vi "Dialog GraphSetting (Chart).vi"(11 "波形チャートref(in)":refnum<vi>) -> ()   [LabVIEW 2014]
uses:
  TypeDef/GraphSetting Appearance.ctl
  TypeDef/GraphSetting Plot.ctl
  SupportVIs/GraphSetting Scale.ctl
  TypeDef/GraphSetting DisplayFormatType.ctl
  TypeDef/GraphSetting All.ctl
  TypeDef/GraphSetting Command.ctl
  Lib/Event/Write User Event (Array).vi
  <vilib>/Utility/xml.llb/Write to XML File(string).vi
  <vilib>/Utility/xml.llb/Read From XML File(string).vi
panel:
  in  "ファイル読込":bool
  in  "ファイル保存":bool
  in  "タブ制御器":enum32{"外観", "スケール", "プロット"}(tab)
  in  "外観":T1
  in  "Yスケール選択":u16(ring) items=["振幅"]
  in  "スケール(Y軸)":T2
  in  "スケール(X軸)":T2
  in  "Xスケール選択":u16(ring) items=["時間"]
  in  "プロット":T4 {"Yスケール" items=["振幅"]; "Xスケール" items=["時間"]; "プロット補間" max=5 step=1; "ポイントスタイル" max=16 step=1; "太さ" max=5 step=1; "ラインスタイル" max=4 step=1}
  in  "プロット選択":u16(ring) items=["正弦波", "プロット1"]
  in  "停止ボタン":bool
  # "欄外、パラメータ"
  # "スケールのスタイルとカラー"
  # "スケール係数"
  # "スケールのスタイルとカラー"
  # "スケールのスタイルとカラー"
  # "スケール係数"
  # "スケールのスタイルとカラー"
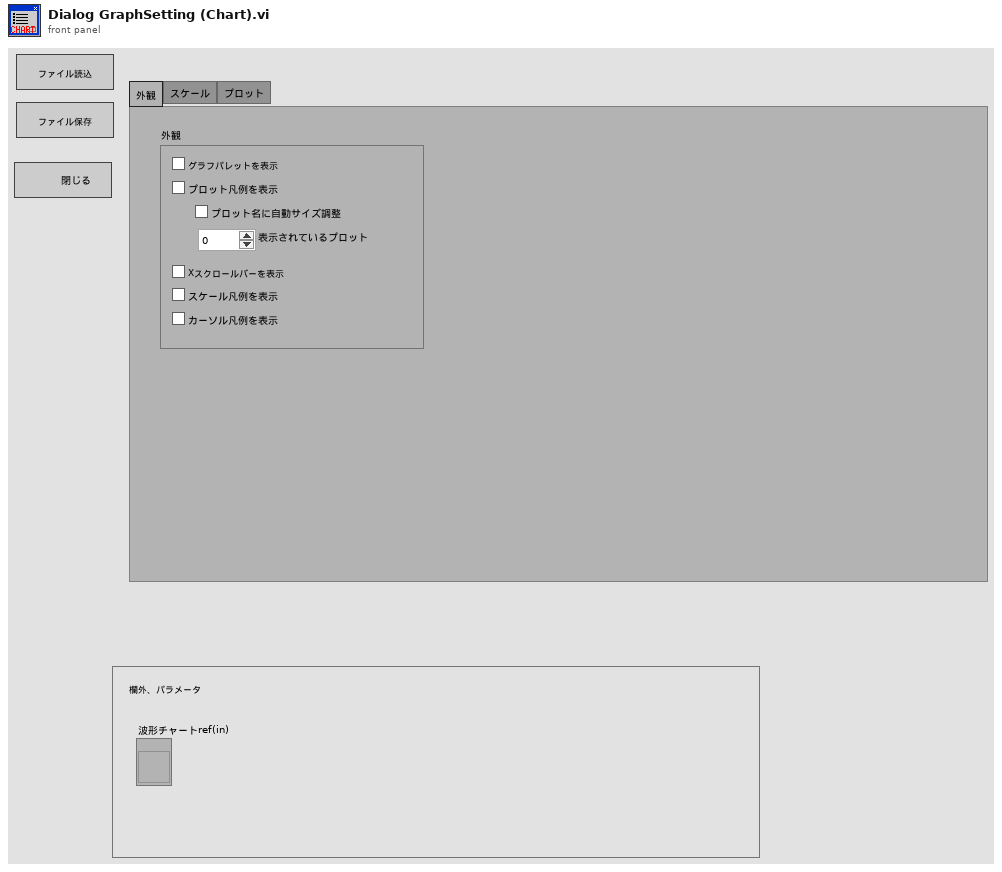
[diagram p1: front panel]
types:
  T1 = typedef "GraphSetting Appearance.ctl" = cluster{"グラフパレットを表示":bool, "プロット凡例を表示":bool, "プロット名に自動サイズ調整":bool, "表示されているプロット":u32, "Xスクロールバーを表示":bool, "スケール凡例を表示":bool, "カーソル凡例を表示":bool}
  T2 = typedef "GraphSetting Scale.ctl" = cluster{"名前":string, "スケールラベルを表示":bool, "スケールを表示":bool, "ログ":bool, "反転":bool, "自動スケール":bool, "最小":dbl, "最大":dbl, "オフセット":dbl, "乗数":dbl, "主目盛り":u32, "補助目盛り":u32, "マーカテキスト":u32, "主グリッド":u32, "補助グリッド":u32, "タイプ":T3, "小数点以下桁数":u8}
  T3 = typedef "GraphSetting DisplayFormatType.ctl" = enum8{"浮動小数点", "科学", "工学", "バイナリ", "８進数", "１６進数", "相対時間", "時間と日時", "SI"}
  T4 = typedef "GraphSetting Plot.ctl" = cluster{"名前":string, "表示":bool, "ラインスタイル":u8, "太さ":u8, "ポイントスタイル":u8, "プロット補間":u8, "ラインカラー":u32, "ポイント/塗りつぶし":u32, "Xスケール":u16, "Yスケール":u16}
  T5 = typedef "GraphSetting All.ctl" = cluster{"外観":T1, "スケールX[]":T2[], "スケールY[]":T2[], "プロット[]":T4[]}
  T6 = typedef "GraphSetting Command.ctl" = enum16{"Get(ref->ctl)", "Set(ctl->ref)"}
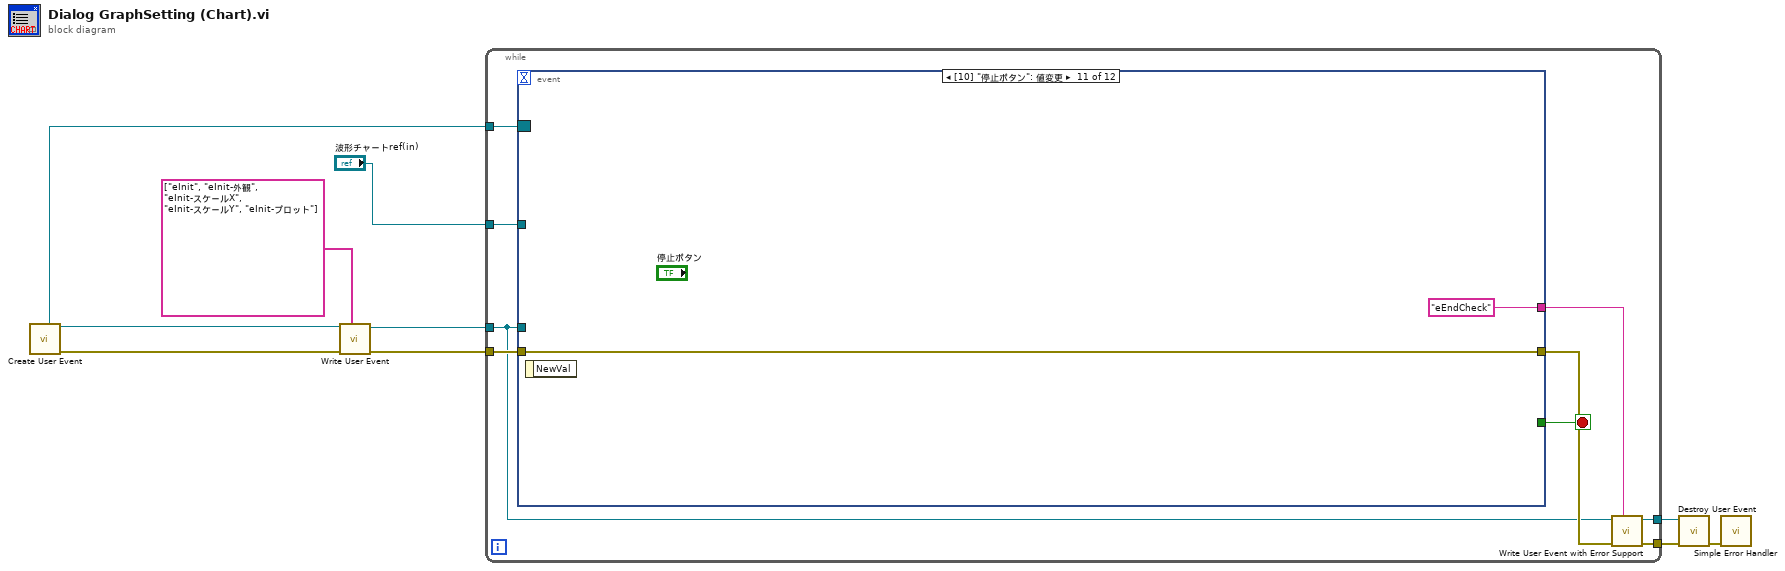
[diagram p0: block diagram]
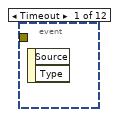
[diagram p2: hidden frame]
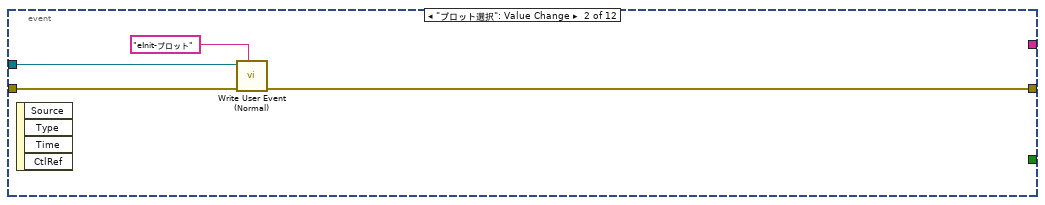
[diagram p3: hidden frame]
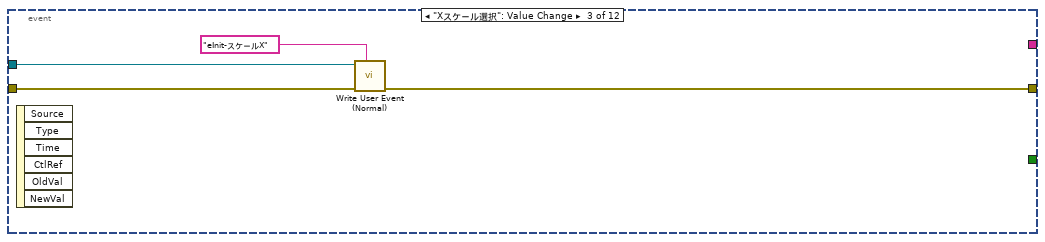
[diagram p4: hidden frame]
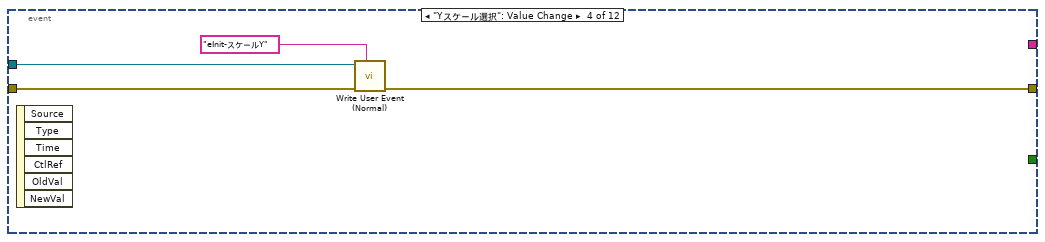
[diagram p5: hidden frame]
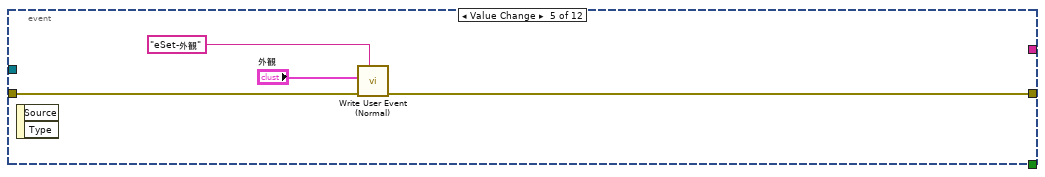
[diagram p6: hidden frame]
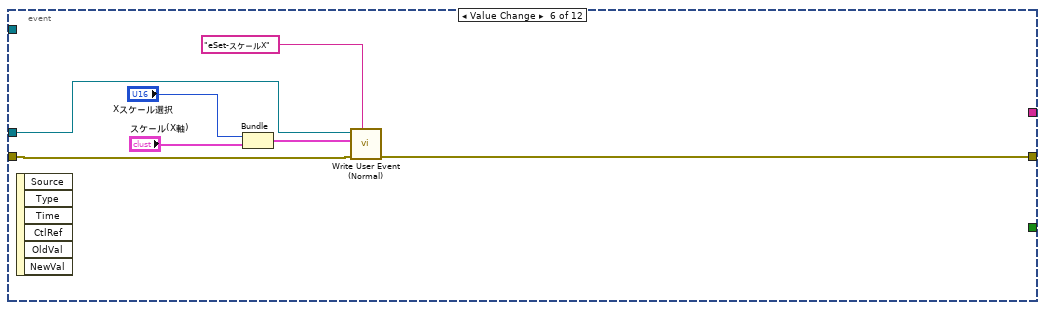
[diagram p7: hidden frame]
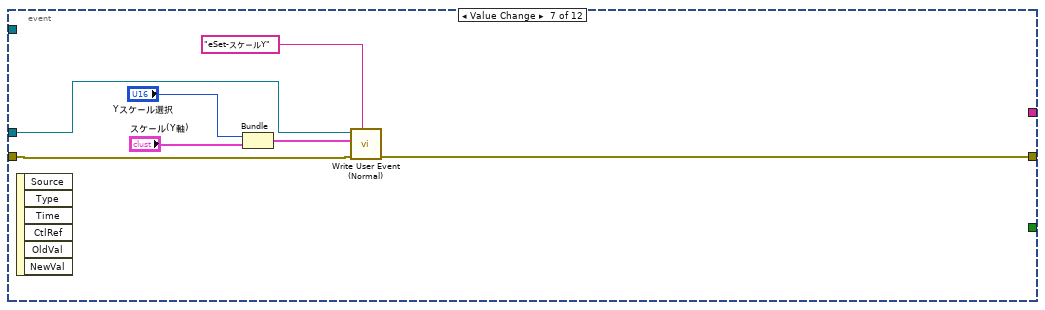
[diagram p8: hidden frame]
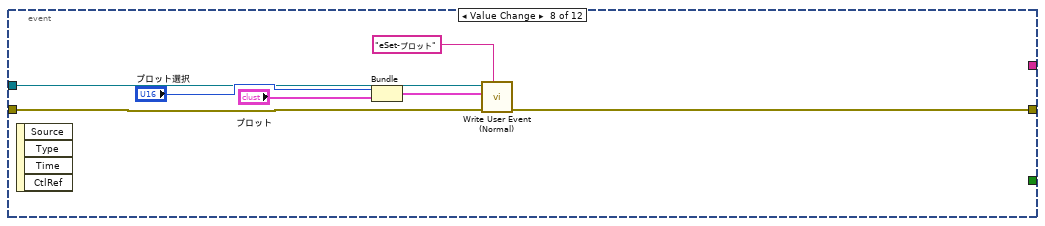
[diagram p9: hidden frame]
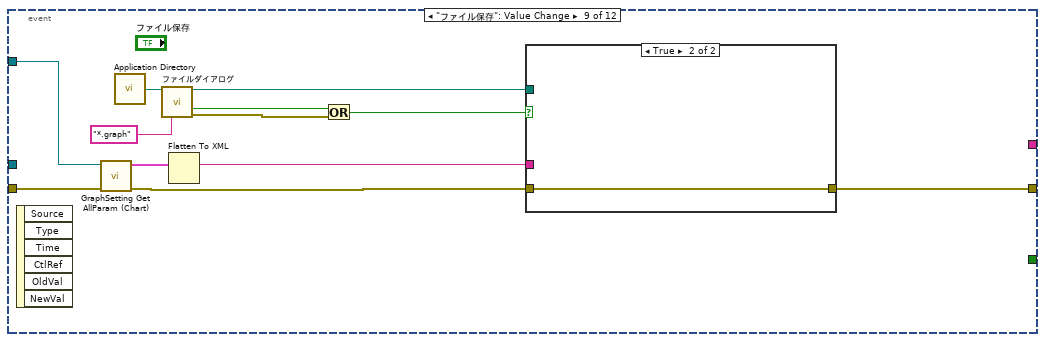
[diagram p10: hidden frame]
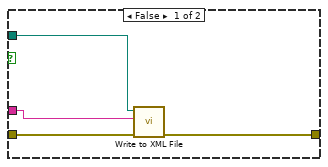
[diagram p11: hidden frame]
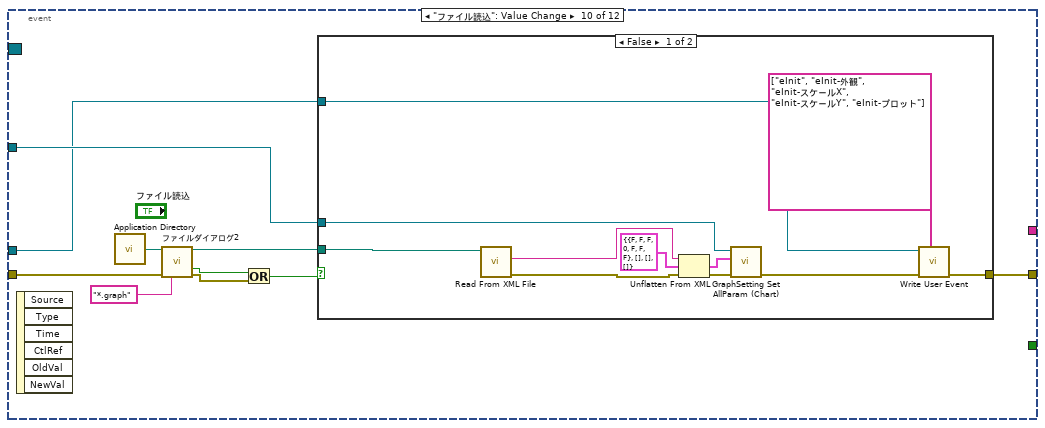
[diagram p12: hidden frame]
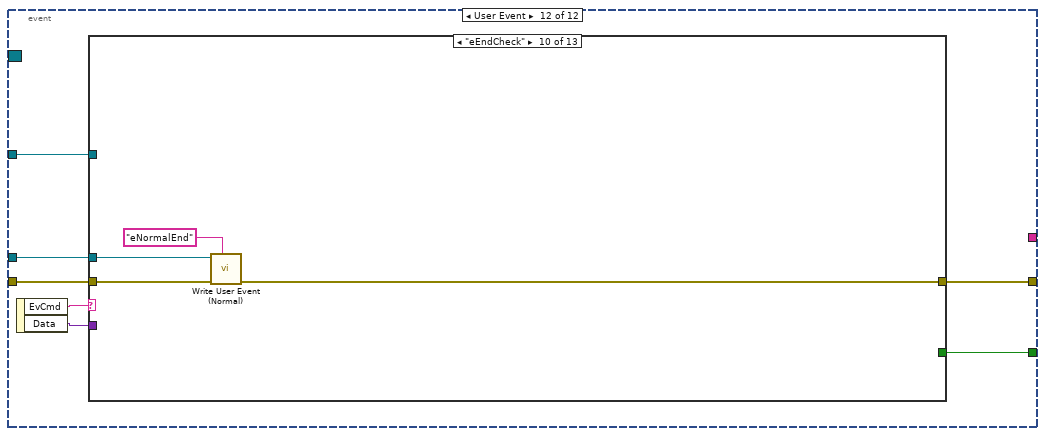
[diagram p14: hidden frame]
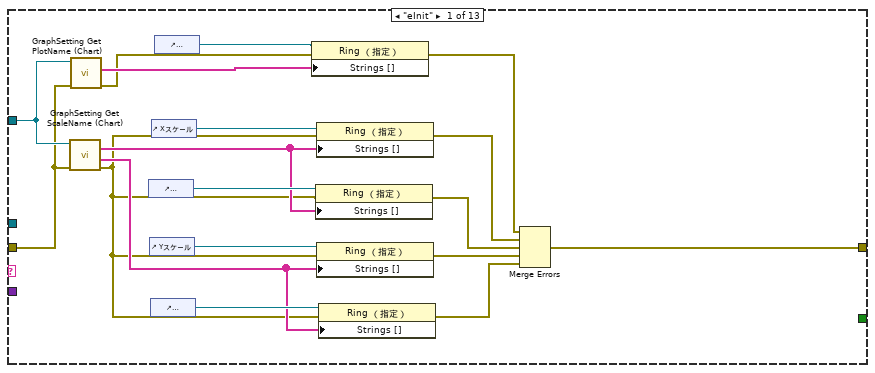
[diagram p15: hidden frame]
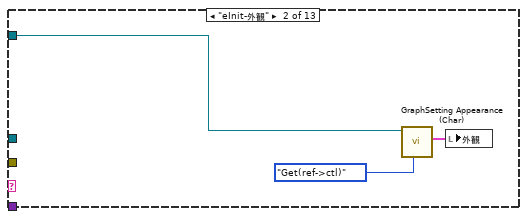
[diagram p16: hidden frame]
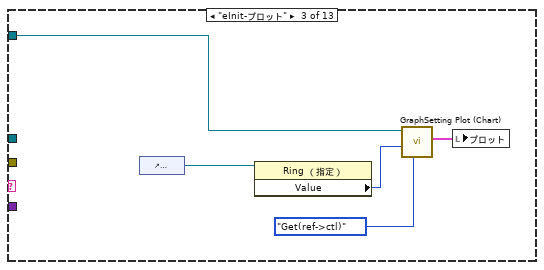
[diagram p17: hidden frame]
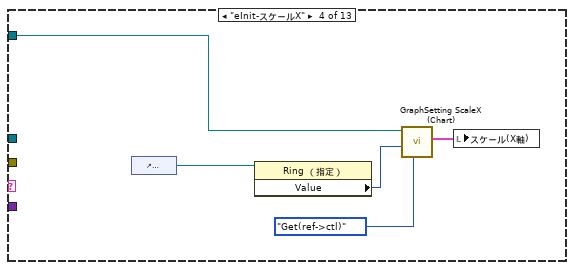
[diagram p18: hidden frame]
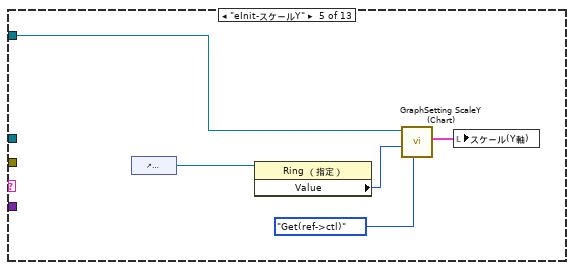
[diagram p19: hidden frame]
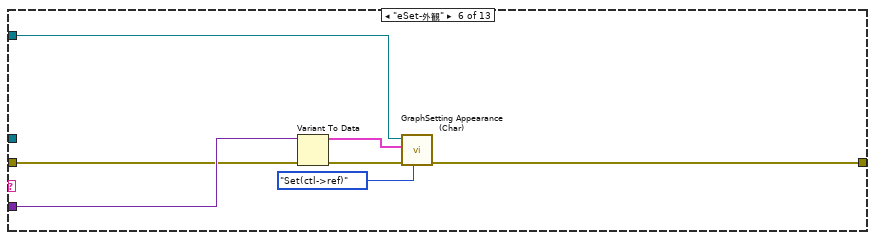
[diagram p20: hidden frame]
diagram:
  n1 = call "Create User Event.vi"() -> ("error out"=w8:errorcluster, "User Event"=w9:refnum<user-event>, "Event Registration Refnum"=w10:refnum<event-registration>)  [unwired: 9 in]
  n2 = call-poly "Write User Event.vi"("EvCmd[]"=string[] ["eInit", "eInit-外観", "eInit-スケールX", "eInit-スケールY", "eInit-プロット"], "エラー入力（エラーなし）"=w8, "ユーザイベント入力"=w9) -> ("エラー出力"=w4:errorcluster, "ユーザイベント出力"=w5:refnum<user-event>)  [unwired: 7 in]
  n3 = while {
    tunnel: w4 -> [w18]
    tunnel: w10 -> [w19]
    tunnel: [w15] -> w7
    tunnel: w5 -> [w11]
    tunnel: "波形チャートref(in)" -> [w17]
    tunnel: [w12] -> w2
    stop <- w13 stop-if-true
    n4 = event shown="[10] \"停止ボタン\": 値変更" {
      selector: w19 -> [_ _ _ _ _ _ _ _ _ _ _ _]
      dyn-events: _ -> [_ _ _ _ _ _ _ _ _ _ _ _]
      timeout: _ -> [_ _ _ _ _ _ _ _ _ _ _ _]
      tunnel: [_ _ _ _ _ _ _ _ _ _ _ w99] -> w13
      tunnel: [_ w21 w25 w28 w32 w37 w44 w51 w60 w78 w95 w100] -> w16
      tunnel: w18 -> [_ w22 w27 w30 w33 w36 w45 w52 w67 w81 w95 w101]
      tunnel: w11 -> [_ w23 w26 w29 _ w40 w46 w53 _ w77 _ w98]
      tunnel: w17 -> [_ _ _ _ _ _ _ _ w68 w79 _ w97]
      tunnel: [_ _ _ _ _ _ _ _ _ _ "eEndCheck" _] -> w14
      event Timeout {
        n5 = event-data() -> ()  [unwired: 1 in, 2 out]
      }
      event "プロット選択": Value Change {
        n6 = event-data() -> ()  [unwired: 1 in, 4 out]
        n7 = call "Write User Event (Normal).vi"("EvCmd"="eInit-プロット", "エラー入力（エラーなし）"=w22, "ユーザイベント入力"=w23) -> ("エラー出力"=w21:errorcluster)  [unwired: 7 in, 1 out]
      }
      event "Xスケール選択": Value Change {
        n8 = event-data() -> ()  [unwired: 1 in, 6 out]
        n9 = call "Write User Event (Normal).vi"("EvCmd"="eInit-スケールX", "エラー入力（エラーなし）"=w27, "ユーザイベント入力"=w26) -> ("エラー出力"=w25:errorcluster)  [unwired: 7 in, 1 out]
      }
      event "Yスケール選択": Value Change {
        n10 = event-data() -> ()  [unwired: 1 in, 6 out]
        n11 = call "Write User Event (Normal).vi"("EvCmd"="eInit-スケールY", "エラー入力（エラーなし）"=w30, "ユーザイベント入力"=w29) -> ("エラー出力"=w28:errorcluster)  [unwired: 7 in, 1 out]
      }
      event Value Change {
        n12 = event-data() -> ()  [unwired: 1 in, 2 out]
        n13 = call "Write User Event (Normal).vi"("EvCmd"="eSet-外観", "エラー入力（エラーなし）"=w33, "データ"="外観") -> ("エラー出力"=w32:errorcluster)  [unwired: 7 in, 1 out]
      }
      event Value Change {
        n14 = event-data() -> ()  [unwired: 1 in, 6 out]
        n15 = Bundle("Xスケール選択"="Xスケール選択", "スケール(X軸)"="スケール(X軸)") -> (w41:cluster{"Xスケール選択":u16, "スケール(X軸)":T2})  [unwired: 1 in]
        n16 = call "Write User Event (Normal).vi"("EvCmd"="eSet-スケールX", "エラー入力（エラーなし）"=w36, "データ"=w41, "ユーザイベント入力"=w40) -> ("エラー出力"=w37:errorcluster)  [unwired: 6 in, 1 out]
      }
      event Value Change {
        n17 = event-data() -> ()  [unwired: 1 in, 6 out]
        n18 = Bundle("Yスケール選択"="Yスケール選択", "スケール(Y軸)"="スケール(Y軸)") -> (w47:cluster{"Yスケール選択":u16, "スケール(Y軸)":T2})  [unwired: 1 in]
        n19 = call "Write User Event (Normal).vi"("EvCmd"="eSet-スケールY", "エラー入力（エラーなし）"=w45, "データ"=w47, "ユーザイベント入力"=w46) -> ("エラー出力"=w44:errorcluster)  [unwired: 6 in, 1 out]
      }
      event Value Change {
        n20 = event-data() -> ()  [unwired: 1 in, 4 out]
        n21 = Bundle("プロット選択"="プロット選択", "プロット"="プロット") -> (w54:cluster{"プロット選択":u16, "プロット":T4})  [unwired: 1 in]
        n22 = call "Write User Event (Normal).vi"("EvCmd"="eSet-プロット", "エラー入力（エラーなし）"=w52, "データ"=w54, "ユーザイベント入力"=w53) -> ("エラー出力"=w51:errorcluster)  [unwired: 6 in, 1 out]
      }
      event "ファイル保存": Value Change {
        n23 = event-data() -> ()  [unwired: 1 in, 6 out]
        n24 = call "GraphSetting Get AllParam (Chart).vi"("エラー入力（エラーなし）"=w67, "WaveformChart入力"=w68) -> ("エラー出力"=w62:errorcluster, "クラスタ"=w61:cluster{"外観(out)":T1, T2[], T2[], T4[]})  [unwired: 8 in]
        n25 = call <vilib>:"Application Directory.vi"() -> ("Application Directory"=w65:path)
        n26 = call "ファイルダイアログ"("start path"=w65, "pattern (all files)"="*.graph") -> ("selected path"=w63:path, "cancelled"=w59:bool, "error out"=w58:errorcluster)  [unwired: 10 in, 1 out]
        n27 = Flatten To XML(anything=w61) -> (xml string=w64:string)
        n28 = Or(x=w59, y=w58) -> (x .or. y?=w57:bool)
        n29 = case shown="TRUE" w57 {
          tunnel: w63 -> [w72 _]
          tunnel: w64 -> [w71 _]
          tunnel: w62 -> [w69 w73]
          tunnel: [w70 w73] -> w60
          frame False {
            n30 = call-poly <vilib>:"Write to XML File.vi"("error in (no error)"=w69, "XML Input"=w71, "XML File Path"=w72) -> ("error out"=w70:errorcluster)  [unwired: 6 in, 2 out]
          }
          frame True {
          }
        }
      }
      event "ファイル読込": Value Change {
        n31 = event-data() -> ()  [unwired: 1 in, 6 out]
        n32 = call <vilib>:"Application Directory.vi"() -> ("Application Directory"=w83:path)
        n33 = call "ファイルダイアログ2"("start path"=w83, "error in"=w81, "pattern (all files)"="*.graph") -> ("selected path"=w80:path, "cancelled"=w75:bool, "error out"=w74:errorcluster)  [unwired: 9 in, 1 out]
        n34 = Or(x=w75, y=w74) -> (x .or. y?=w76:bool)
        n35 = case shown="FALSE" w76 {
          tunnel: w80 -> [w92 _]
          tunnel: w79 -> [w88 _]
          tunnel: [w85 _] -> w78
          tunnel: w77 -> [w87 _]
          frame False {
            n36 = call-poly <vilib>:"Read From XML File.vi"("XML File Path"=w92) -> ("error out"=w91:errorcluster, "XML Elements"=w93:string)  [unwired: 8 in, 1 out]
            n37 = Unflatten From XML(xml string=w93, type=T5 {"外観"={"グラフパレットを表示"=FALSE, "プロット凡例を表示"=FALSE, "プロット名に自動サイズ調整"=FALSE, "表示されているプロット"=0, "Xスクロールバーを表示"=FALSE, "スケール凡例を表示"=FALSE, "カーソル凡例を表示"=FALSE}, "スケールX[]"=[], "スケールY[]"=[], "プロット[]"=[]} ("出力クラスタ"), error in (no error)=w91) -> (value=w90:T5, error out=w89:errorcluster)
            n38 = call "GraphSetting Set AllParam (Chart).vi"("error in (no error)"=w89, "Chartグラフパラメータ"=w90, "波形チャートref(in)"=w88) -> ("error out"=w86:errorcluster)  [unwired: 8 in]
            n39 = call-poly "Write User Event.vi"("EvCmd[]"=string[] ["eInit", "eInit-外観", "eInit-スケールX", "eInit-スケールY", "eInit-プロット"], "エラー入力（エラーなし）"=w86, "ユーザイベント入力"=w87) -> ("エラー出力"=w85:errorcluster)  [unwired: 7 in, 1 out]
          }
          frame True {
          }
        }
      }
      event "停止ボタン": Value Change {
        n40 = event-data() -> ()  [unwired: 1 in, 1 out]
      }
      event User Event {
        n41 = event-data() -> ("EvCmd"=w103:string, "Data"=w102:variant)  [unwired: 1 in]
        n42 = case shown="\"eEndCheck\"" w103 {
          selector: w103 -> [_ _ _ _ _ _ _ _ _ _ _ _ w187]
          tunnel: w102 -> [_ _ _ _ _ w144 w152 w163 w173 _ _ w186 _]
          tunnel: w101 -> [w113 _ _ _ _ w142 w154 w162 w172 w177 w181 w184 _]
          tunnel: [w104 _ _ _ _ w140 w147 w156 w166 w176 w181 _ _] -> w100
          tunnel: [_ _ _ _ _ _ _ _ _ _ TRUE TRUE _] -> w99
          tunnel: w98 -> [_ _ _ _ _ _ _ _ _ w179 _ _ _]
          tunnel: w97 -> [w116 w124 w129 w134 w139 w145 w148 w160 w170 _ _ _ _]
          frame "eInit" {
            n43 = call "GraphSetting Get ScaleName (Chart).vi"("error in (no error)"=w113, "波形チャートref(in)"=w116) -> ("error out"=w110:errorcluster, "Y軸名称[]"=w112:string[], "X軸名称[]"=w119:string[])  [unwired: 7 in]
            n44 = call "GraphSetting Get PlotName (Chart).vi"("error in (no error)"=w113, "波形チャートref(in)"=w116) -> ("error out"=w111:errorcluster, "プロット名称[]"=w114:string[])  [unwired: 8 in]
            n45 = control-ref of="Xスケール選択"() -> (w120:refnum<vi>)
            n46 = control-ref of="Yスケール"() -> (w117:refnum<vi>)
            n47 = control-ref of="Yスケール選択"() -> (w118:refnum<vi>)
            n48 = control-ref of="Xスケール"() -> (w121:refnum<vi>)
            n49 = control-ref of="プロット選択"() -> (w115:refnum<vi>)
            n50 = property class="Ring （指定）"(reference=w115, error in=w111, "Strings []"=w114) -> (error out=w109:errorcluster)  [unwired: 1 out]
            n51 = property class="Ring （指定）"(reference=w120, error in=w110, "Strings []"=w119) -> (error out=w107:errorcluster)  [unwired: 1 out]
            n52 = property class="Ring （指定）"(reference=w121, error in=w110, "Strings []"=w119) -> (error out=w108:errorcluster)  [unwired: 1 out]
            n53 = property class="Ring （指定）"(reference=w117, error in=w110, "Strings []"=w112) -> (error out=w106:errorcluster)  [unwired: 1 out]
            n54 = property class="Ring （指定）"(reference=w118, error in=w110, "Strings []"=w112) -> (error out=w105:errorcluster)  [unwired: 1 out]
            n55 = Merge Errors(w109, w108, w107, w106, w105) -> (w104:errorcluster)
          }
          frame "eInit-外観" {
            n56 = call "GraphSetting Appearance (Char).vi"("コマンド"=GraphSetting_Command."Get(ref->ctl)", "WaveformChart入力"=w124) -> ("外観(out)"=w123:T1)  [unwired: 8 in, 1 out]
            n57 = local write "外観"(w123) -> ()
          }
          frame "eInit-プロット" {
            n58 = control-ref of="プロット選択"() -> (w128:refnum<vi>)
            n59 = property class="Ring （指定）"(reference=w128) -> ("Value"=w127:u16)  [unwired: 1 in, 2 out]
            n60 = call "GraphSetting Plot (Chart).vi"("コマンド"=GraphSetting_Command."Get(ref->ctl)", "アクティブプロット"=w127, "波形チャートref(in)"=w129) -> ("プロット(out)"=w125:T4)  [unwired: 7 in, 1 out]
            n61 = local write "プロット"(w125) -> ()
          }
          frame "eInit-スケールX" {
            n62 = control-ref of="Xスケール選択"() -> (w133:refnum<vi>)
            n63 = property class="Ring （指定）"(reference=w133) -> ("Value"=w132:u16)  [unwired: 1 in, 2 out]
            n64 = call "GraphSetting ScaleX (Chart).vi"("コマンド"=GraphSetting_Command."Get(ref->ctl)", "アクティブスケール(X)"=w132, "波形チャートref(in)"=w134) -> ("スケール(out)"=w130:T2)  [unwired: 7 in, 1 out]
            n65 = local write "スケール(X軸)"(w130) -> ()
          }
          frame "eInit-スケールY" {
            n66 = control-ref of="Yスケール選択"() -> (w138:refnum<vi>)
            n67 = property class="Ring （指定）"(reference=w138) -> ("Value"=w137:u16)  [unwired: 1 in, 2 out]
            n68 = call "GraphSetting ScaleY (Chart).vi"("コマンド"=GraphSetting_Command."Get(ref->ctl)", "アクティブスケールY"=w137, "波形チャートref(in)"=w139) -> ("スケール(out)"=w135:T2)  [unwired: 7 in, 1 out]
            n69 = local write "スケール(Y軸)"(w135) -> ()
          }
          frame "eSet-外観" {
            n70 = Variant To Data(error in=w142, Variant=w144) -> (data=w143:T1, error out=w141:errorcluster)  [unwired: 1 in]
            n71 = call "GraphSetting Appearance (Char).vi"("コマンド"=GraphSetting_Command."Set(ctl->ref)", "error in (no error)"=w141, "外観(in)"=w143, "WaveformChart入力"=w145) -> ("error out"=w140:errorcluster)  [unwired: 6 in, 1 out]
          }
          frame "eSet-スケールX" {
            n72 = Variant To Data(type=cluster{"Xスケール選択":u16, "スケール(X軸)":T2} {"Xスケール選択"=0, "スケール(X軸)"={"名前"="", "スケールラベルを表示"=FALSE, "スケールを表示"=FALSE, "ログ"=FALSE, "反転"=FALSE, "自動スケール"=FALSE, "最小"=0.0, "最大"=0.0, "オフセット"=0.0, "乗数"=0.0, "主目盛り"=0, "補助目盛り"=0, "マーカテキスト"=0, "主グリッド"=0, "補助グリッド"=0, "タイプ"=enum."浮動小数点", "小数点以下桁数"=0}} ("出力クラスタ"), Variant=w152) -> (data=w151:cluster{"Xスケール選択":u16, "スケール(X軸)":T2})  [unwired: 1 in, 1 out]
            n73 = Unbundle(w151) -> ("Xスケール選択"=w149:u16, "スケール(X軸)"=w150:T2)
            n74 = call "GraphSetting ScaleX (Chart).vi"("コマンド"=GraphSetting_Command."Set(ctl->ref)", "error in (no error)"=w154, "アクティブスケール(X)"=w149, "スケール(in)"=w150, "波形チャートref(in)"=w148) -> ("error out"=w147:errorcluster)  [unwired: 5 in, 1 out]
          }
          frame "eSet-スケールY" {
            n75 = Variant To Data(error in=w162, type=cluster{"Xスケール選択":u16, "スケール(X軸)":T2} {"Xスケール選択"=0, "スケール(X軸)"={"名前"="", "スケールラベルを表示"=FALSE, "スケールを表示"=FALSE, "ログ"=FALSE, "反転"=FALSE, "自動スケール"=FALSE, "最小"=0.0, "最大"=0.0, "オフセット"=0.0, "乗数"=0.0, "主目盛り"=0, "補助目盛り"=0, "マーカテキスト"=0, "主グリッド"=0, "補助グリッド"=0, "タイプ"=enum."浮動小数点", "小数点以下桁数"=0}} ("出力クラスタ"), Variant=w163) -> (data=w161:cluster{"Xスケール選択":u16, "スケール(X軸)":T2}, error out=w157:errorcluster)
            n76 = Unbundle(w161) -> ("Xスケール選択"=w158:u16, "スケール(X軸)"=w159:T2)
            n77 = call "GraphSetting ScaleY (Chart).vi"("コマンド"=GraphSetting_Command."Set(ctl->ref)", "error in (no error)"=w157, "アクティブスケールY"=w158, "スケール(in)"=w159, "波形チャートref(in)"=w160) -> ("error out"=w156:errorcluster)  [unwired: 5 in, 1 out]
          }
          frame "eSet-プロット" {
            n78 = Variant To Data(error in=w172, type=cluster{"プロット選択":u16, "プロット":T4} {"プロット選択"=0, "プロット"={"名前"="", "表示"=FALSE, "ラインスタイル"=0, "太さ"=0, "ポイントスタイル"=0, "プロット補間"=0, "ラインカラー"=0, "ポイント/塗りつぶし"=0, "Xスケール"=0, "Yスケール"=0}} ("出力クラスタ"), Variant=w173) -> (data=w171:cluster{"プロット選択":u16, "プロット":T4}, error out=w169:errorcluster)
            n79 = Unbundle(w171) -> ("プロット選択"=w168:u16, "プロット"=w167:T4)
            n80 = call "GraphSetting Plot (Chart).vi"("コマンド"=GraphSetting_Command."Set(ctl->ref)", "error in (no error)"=w169, "アクティブプロット"=w168, "プロット(in)"=w167, "波形チャートref(in)"=w170) -> ("error out"=w166:errorcluster)  [unwired: 5 in, 1 out]
          }
          frame "eEndCheck" {
            n81 = call "Write User Event (Normal).vi"("EvCmd"="eNormalEnd", "エラー入力（エラーなし）"=w177, "ユーザイベント入力"=w179) -> ("エラー出力"=w176:errorcluster)  [unwired: 7 in, 1 out]
          }
          frame "eNormalEnd" {
          }
          frame "eErrorEnd" {
            n82 = Variant To Data(error in=w184, type=errorcluster {"status"=FALSE, "code"=0, "source"=""} ("エラー定数"), Variant=w186) -> (data=w183:errorcluster)  [unwired: 1 out]
            n83 = call <vilib>:"Simple Error Handler.vi"("error in (no error)"=w183) -> ()  [unwired: 4 in, 5 out]
          }
          frame Default {
            n84 = call "DialogProgramError.vi"("エラー内容"="ユーザイベント例外" ("エラー詳細"), "エラー詳細"=w187) -> ()  [unwired: 9 in, 1 out]
          }
        }
      }
    }
    n85 = call "Write User Event with Error Support.vi"("EvCmd"=w14, "エラー入力（エラーなし）"=w16, "ユーザイベント入力"=w11) -> ("エラー出力"=w15:errorcluster, "ユーザイベント出力"=w12:refnum<user-event>)  [unwired: 7 in]
  }
  n86 = call "Destroy User Event.vi"("error in (no error)"=w7, "User Event"=w2) -> ("error out"=w6:errorcluster)  [unwired: 9 in]
  n87 = call <vilib>:"Simple Error Handler.vi"("error in (no error)"=w6) -> ()  [unwired: 4 in, 5 out]
